vi "Get Directories.vi"(8 "error in (no error)":errorcluster caption="错误输入（无错误）", 10 "Directory":path) -> (0 "error out":errorcluster caption="错误输出", 2 "Directories":path[](array[path]))   [LabVIEW 2012, in "Directory.lvclass"]
uses:
  Directory.lvclass
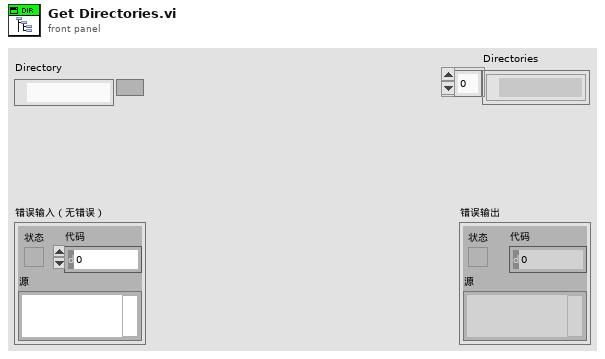
[diagram p1: front panel]
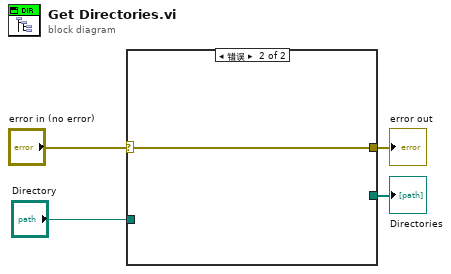
[diagram p0: block diagram]
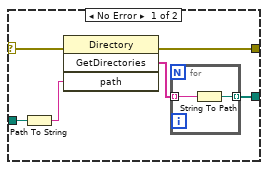
[diagram p2: hidden frame]
diagram:
  n1 = case shown="错误" "error in (no error)" {
    selector: "error in (no error)" -> [w10 w13]
    tunnel: [w9 w13] -> w3
    tunnel: "Directory" -> [w8 _]
    tunnel: [w5 _] -> w1
    frame No Error {
      n2 = Path To String(path=w8) -> (string=w7:string)
      n3 = invoke on="调用节点" class="Directory" method="GetDirectories"(error in=w10, "path"=w7) -> (error out=w9:errorcluster, "GetDirectories"=w6:string[])  [unwired: 2 in, 2 out]
      n4 = for {
        tunnel: w6 -> [w12] mode=indexing
        tunnel: [w11] -> w5 mode=indexing
        n5 = String To Path(string=w12) -> (path=w11:path)
      }
    }
    frame Error {
    }
  }
  "error out" <- w3
  "Directories" <- w1
